vi "myRIO v1.0 DO Block Write.vi"(5 "Wait Until Done?":bool, 6 "DO FIFO Sample Rate (Hz)":dbl=1000.0 min=1000.0 max=8000000.0, 8 "error in (no error)":errorcluster, 9 "bool Value List":bool[][](array[boolean]), 10 "DO (N Samples) Channel List":T3, 11 "myRIO Ref In":T1) -> (0 "error out":errorcluster, 3 "myRIO Ref Out":T1)   [LabVIEW 2021]
uses:
  <vilib>/myRIO/Common/Instrument Driver Framework/myRIO v1.0/DO Block/typedefs/DO Block Channels List.ctl
  <vilib>/myRIO/Common/Instrument Driver Framework/myRIO v1.0/DO Block/typedefs/DO Block Channels Enum.ctl
  <vilib>/myRIO/Common/Instrument Driver Framework/Utilities/typedefs/myRIO v1.0 Reference.ctl
  <vilib>/myRIO/Common/Instrument Driver Framework/Utilities/typedefs/Generic FPGA Reference.ctl
  <vilib>/myRIO/Common/Instrument Driver Framework/myRIO v1.0/DO Block/typedefs/DO Block FPGA Reference.ctl
  <vilib>/myRIO/Common/Instrument Driver Framework/myRIO v1.0/DO Block/typedefs/DO Block Configuration.ctl
  <vilib>/myRIO/Common/Instrument Driver Framework/myRIO v1.0/Resource Manager/vis/myRIO v1.0 Block Write Configuration.vi
  <vilib>/rvi/errors/niLvFpgaAdjustHostInterfaceError.vi
  <vilib>/RVI Host/nirviSupport.llb/nirviErrorClusterFromErrorCode.vi
  <vilib>/rvi/interface/nirviReadWriteControl/nirviReadWriteControl.xnode
  <vilib>/rvi/interface/nirviMethod/nirviMethod.xnode
  <vilib>/rvi/interface/Simulation/niFpgaSimulationCallBeginRW.vi
  <vilib>/rvi/interface/nirviMethod/StockFPGA_InlinedMethodWaitForSingleIRQ.vi
  <vilib>/FPGAPlugInAG/Dynamic/niLvFpga_WaitOnIrq_Dynamic.vi
  <vilib>/FPGAPlugInAG/Dynamic/niLvFpga_AcknowledgeIrq_Dynamic.vi
  NiFpgaLv.dll
  <vilib>/FPGAPlugInAG/Dynamic/niLvFpga_WriteFifo_Dynamic.vi
  <vilib>/rvi/errors/niLvFpgaMergeErrorWithErrorCode.vi
panel:
  # "This VI writes boolean values to user specified a list of DIO channels on the myRIO v1.0 hardware. The values are input as boolean values. Please see Block Diagram for details."
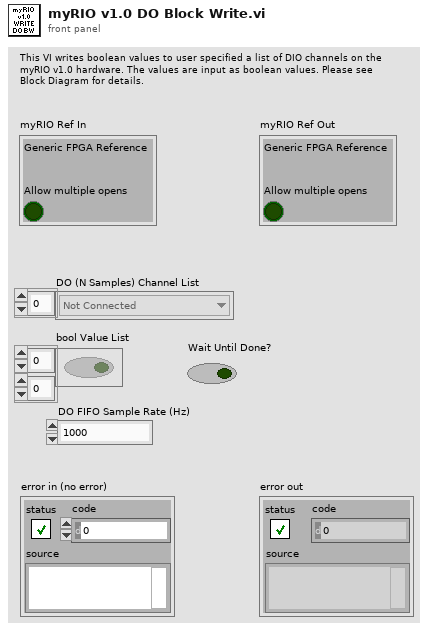
[diagram p1: front panel]
types:
  T1 = typedef "myRIO v1.0 Reference.ctl" = cluster{"Generic FPGA Reference":T2, "Allow multiple opens":bool}
  T2 = typedef "Generic FPGA Reference.ctl" = refnum<k20>
  T3 = typedef "DO Block Channels List.ctl" = T4[]
  T4 = typedef "DO Block Channels Enum.ctl" = enum16{"Not Connected", "A/DO0 (N Samples)", "A/DO1 (N Samples)", "A/DO2 (N Samples)", "A/DO3 (N Samples)", "A/DO4 (N Samples)", "A/DO5 (N Samples)", "A/DO6 (N Samples)", "A/DO7 (N Samples)", "A/DO8 (N Samples)", "A/DO9 (N Samples)", "A/DO10 (N Samples)", "A/DO11 (N Samples)", "A/DO12 (N Samples)", "A/DO13 (N Samples)", "A/DO14 (N Samples)", "A/DO15 (N Samples)", "A/DO16 (N Samples)", "A/DO17 (N Samples)", "A/DO18 (N Samples)", "A/DO19 (N Samples)", "B/DO0 (N Samples)", "B/DO1 (N Samples)", "B/DO2 (N Samples)", "B/DO3 (N Samples)", "B/DO4 (N Samples)", "B/DO5 (N Samples)", "B/DO6 (N Samples)", "B/DO7 (N Samples)", "B/DO8 (N Samples)", "B/DO9 (N Samples)", "B/DO10 (N Samples)", "B/DO11 (N Samples)", "B/DO12 (N Samples)", "B/DO13 (N Samples)", "B/DO14 (N Samples)", "B/DO15 (N Samples)", "B/DO16 (N Samples)", "B/DO17 (N Samples)", "B/DO18 (N Samples)", "B/DO19 (N Samples)"}
  T5 = typedef "DO Block FPGA Reference.ctl" = refnum<k20>
  T6 = typedef "DO Block Configuration.ctl" = cluster{"Wait Until Done?":bool, "DO FIFO Clock Divisor":u16, "Occurrence Handler":refnum<k4>, "Digital data reference":refnum<data-value>}
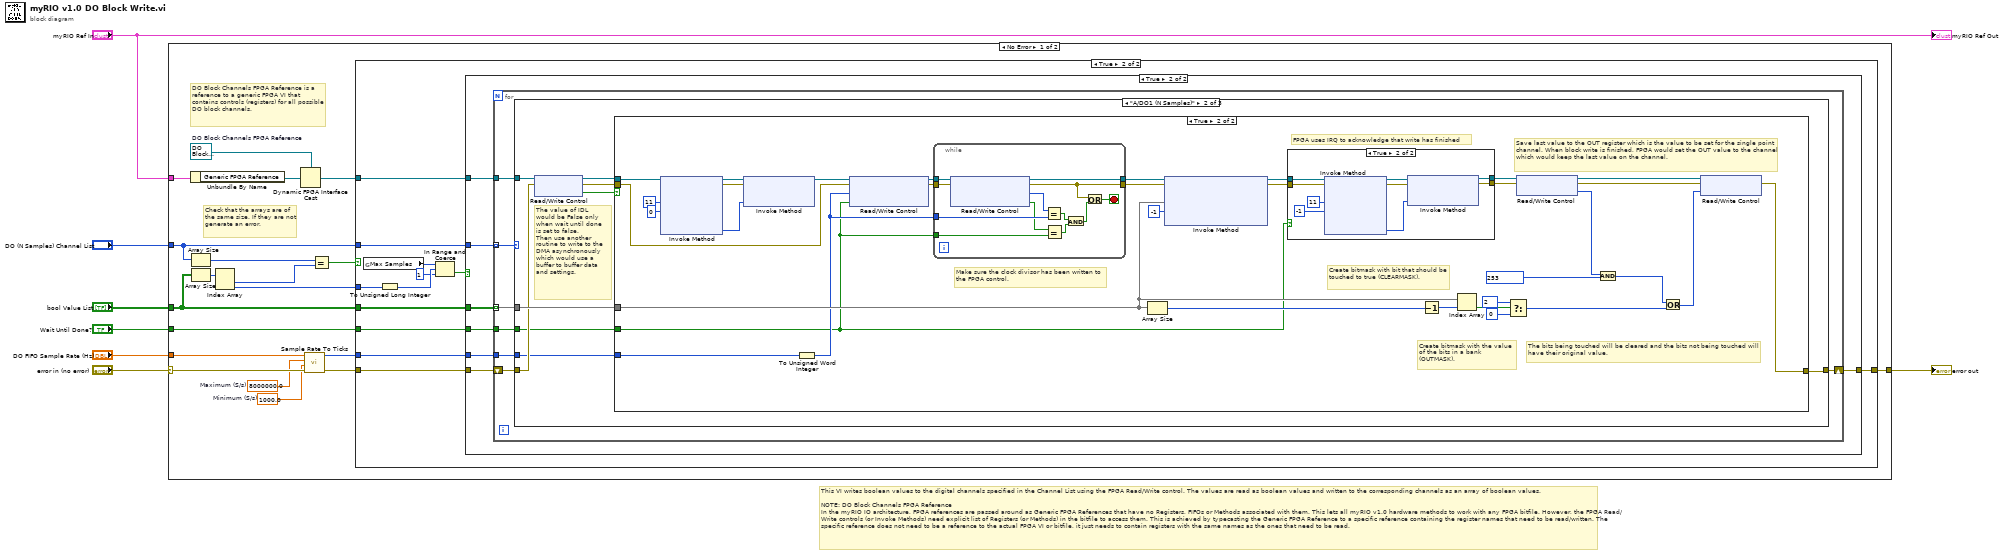
[diagram p0: block diagram]
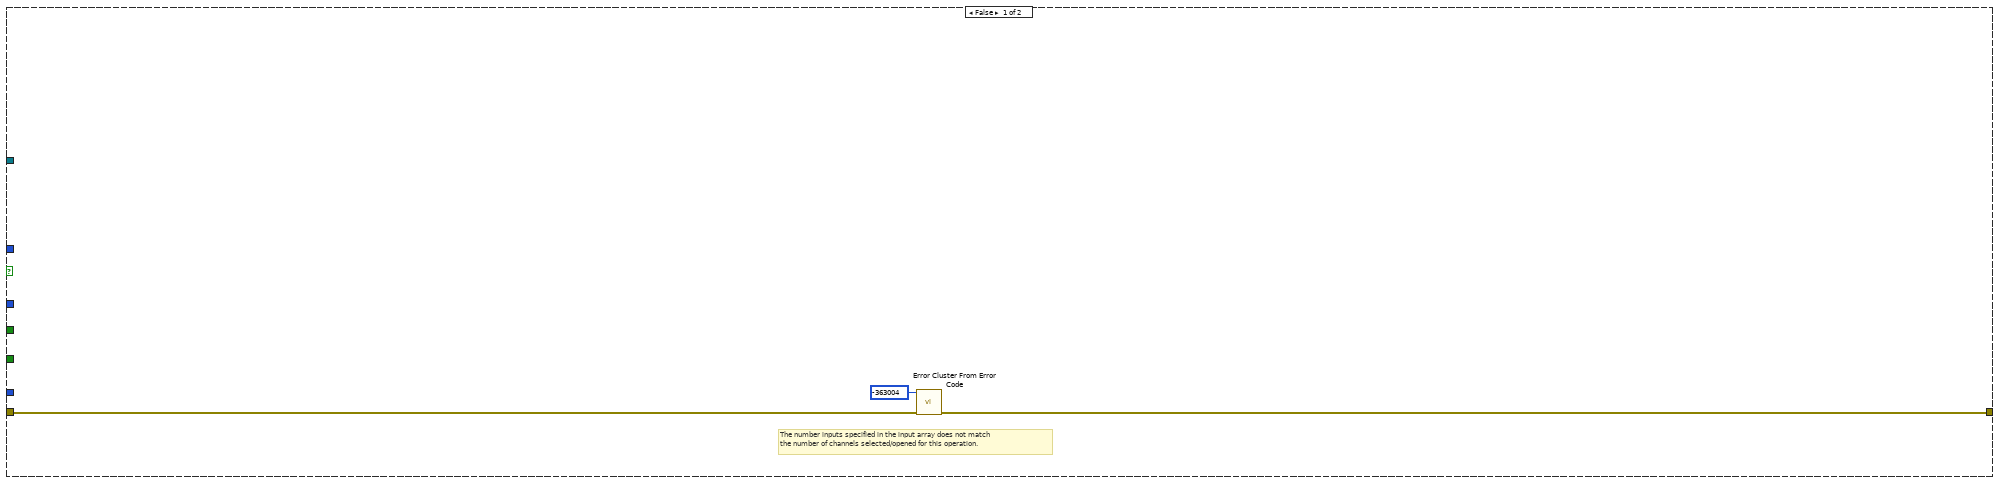
[diagram p2: hidden frame]
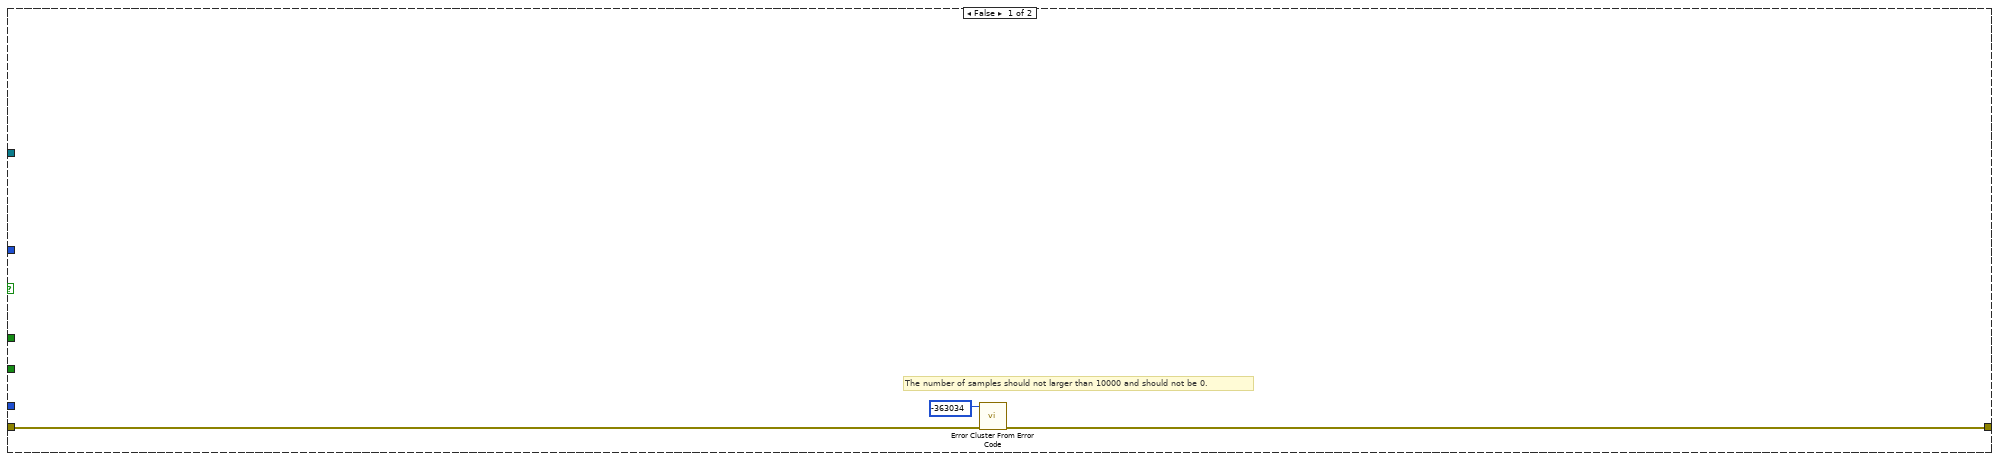
[diagram p3: hidden frame]
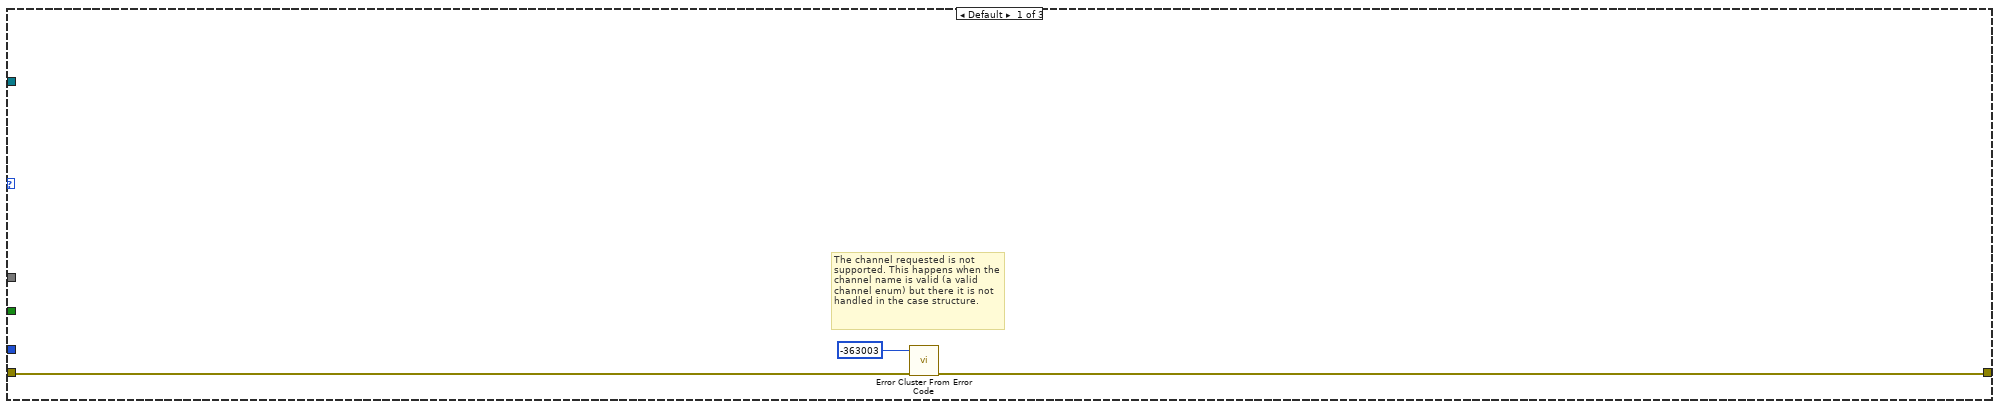
[diagram p4: hidden frame]
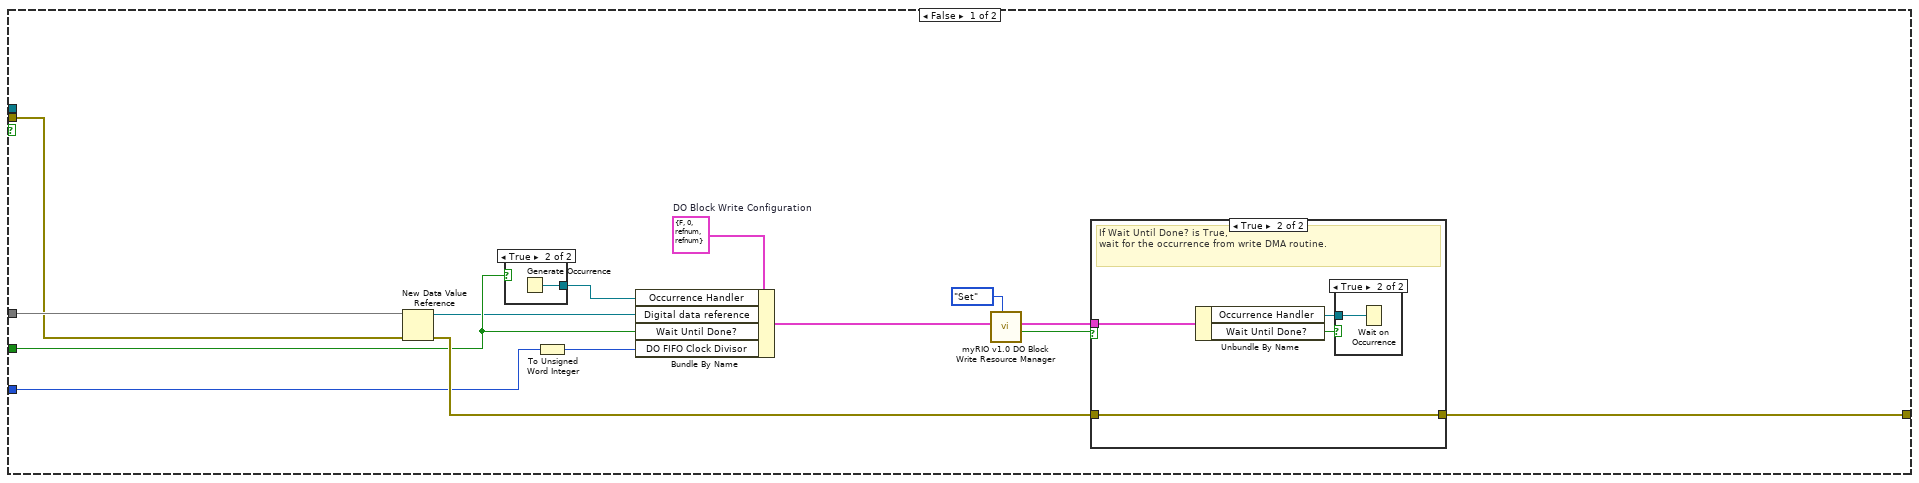
[diagram p5: hidden frame]
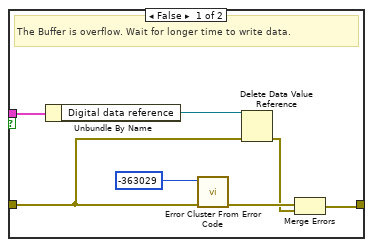
[diagram p6: hidden frame]
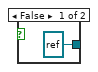
[diagram p8: hidden frame]
diagram:
  # "This VI writes boolean values to the digital channels specified in the Channel List using the FPGA Read/Write control. The values are read as boolean values and written to the corresponding channels as an array of boolean values. \n\nNOTE: DO Block Channels FPGA Reference\nIn the myRIO IO architecture, FPGA references are passed around as Generic FPGA References that have no Registers, FIFOs or Methods associated with them. This lets all myRIO v1.0 hardware methods to work with any FPGA bitfile. However, the FPGA Read/Write controls (or Invoke Methods) need explicit list of Registers (or Methods) in the bitfile to access them. This is achieved by typecasting the Generic FPGA Reference to a specific reference containing the register names that need to be read/written. The specific reference does not need to be a reference to the actual FPGA VI or bitfile, it just needs to contain registers with the same names as the ones that need to be read."
  n1 = case shown="No Error" "error in (no error)" {
    selector: "error in (no error)" -> [w10 w157]
    tunnel: "myRIO Ref In" -> [w26 _]
    tunnel: [w25 w157] -> w6
    tunnel: "DO (N Samples) Channel List" -> [w23 _]
    tunnel: "bool Value List" -> [w22 _]
    tunnel: "DO FIFO Sample Rate (Hz)" -> [w11 _]
    tunnel: "Wait Until Done?" -> [w18 _]
    frame No Error {
      w8 = 1000.0  # Minimum (S/s)
      w9 = 8000000.0  # Maximum (S/s)
      w17 = T5 refnum  # DO Block Channels FPGA Reference
      # "DO Block Channels FPGA Reference is a reference to a generic FPGA VI that contains controls (registers) for all possible DO block channels."
      # "Check that the arrays are of the same size. If they are not generate an error."
      n2 = Unbundle By Name(w26) -> ("Generic FPGA Reference"=w16:T2)
      n3 = Array Size(array=w23) -> (size(s)=w24:i32)
      n4 = Array Size(array=w22) -> (size(s)=w20:i32[])
      n5 = Index Array(array=w20) -> (element #1=w19:i32, element #2=w14:i32)  [unwired: 2 in]
      n6 = Dynamic FPGA Interface Cast(Session In=w17, Type=w16) -> (Session Out=w15:T5)
      n7 = call <vilib>:"Sample Rate To Ticks.vi"("error in (no error)"=w10, "Minimum (S/s)"=w8, "Maximum (S/s)"=w9, "Sample Rate (S/s)"=w11) -> ("error out"=w12:errorcluster, "Count (tick/s)"=w13:u32)  [unwired: 5 in, 1 out]
      n8 = Equal?(x=w24, y=w19) -> (x = y?=w21:bool)
      n9 = case shown="True" w21 {
        tunnel: w23 -> [_ w39]
        tunnel: w22 -> [_ w37]
        tunnel: w12 -> [w28 w41]
        tunnel: [w27 w40] -> w25
        tunnel: w13 -> [_ w38]
        tunnel: w18 -> [_ w34]
        tunnel: w15 -> [_ w36]
        tunnel: w14 -> [_ w35]
        frame False {
          # "The number inputs specified in the input array does not match\nthe number of channels selected/opened for this operation."
          n10 = call <vilib>:"Error Cluster From Error Code.vi"("error in (no error)"=w28, "error code (0)"=-363004) -> ("error out"=w27:errorcluster)  [unwired: 7 in]
        }
        frame True {
          n11 = global read "myRIO v1.0 Block Write Configuration.vi" "Max Samples"() -> (w32:u32)
          n12 = To Unsigned Long Integer(number=w35) -> (unsigned 32bit integer=w31:u32)
          n13 = In Range and Coerce(upper limit=w32, x=w31, lower limit=u32 1) -> (In Range?=w33:bool)  [unwired: 1 out]
          n14 = case shown="True" w33 {
            tunnel: w41 -> [w43 w51]
            tunnel: [w42 w50] -> w40
            tunnel: w39 -> [_ w49]
            tunnel: w38 -> [_ w48]
            tunnel: w37 -> [_ w47]
            tunnel: w36 -> [_ w46]
            tunnel: w34 -> [_ w45]
            frame False {
              # "The number of samples should not larger than 10000 and should not be 0."
              n15 = call <vilib>:"Error Cluster From Error Code.vi"("error in (no error)"=w43, "error code (0)"=-363034) -> ("error out"=w42:errorcluster)  [unwired: 7 in]
            }
            frame True {
              n16 = for {
                tunnel: w46 -> [w57]
                shift-right: [w53] -> w50
                shift-left: w51 -> [w56]
                tunnel: w49 -> [w58] mode=indexing
                tunnel: w48 -> [w55]
                tunnel: w47 -> [w54] mode=indexing
                tunnel: w45 -> [w52]
                n17 = case shown="\"A/DO1 (N Samples)\"" w58 {
                  tunnel: w57 -> [_ w66 _]
                  tunnel: w56 -> [w60 w65 w156]
                  tunnel: w55 -> [_ w62 _]
                  tunnel: w54 -> [_ w67 _]
                  tunnel: [w59 w64 w156] -> w53
                  tunnel: w52 -> [_ w63 _]
                  frame Default {
                    # "The channel requested is not supported. This happens when the channel name is valid (a valid channel enum) but there it is not handled in the case structure."
                    n18 = call <vilib>:"Error Cluster From Error Code.vi"("error in (no error)"=w60, "error code (0)"=-363003) -> ("error out"=w59:errorcluster)  [unwired: 7 in]
                  }
                  frame "A/DO1 (N Samples)" {
                    # "The value of IDL\nwould be False only \nwhen wait until done\nis set to false.\nThen use another \nroutine to write to the \nDMA asynchronously\nwhich would use a \nbuffer to buffer data \nand settings."
                    n19 = xnode "Read/Write Control"("FPGA VI Reference In"=w66, "error in"=w65) -> ("FPGA VI Reference Out"=w70:T5, "error out"=w69:errorcluster, "DO.A_1.IDL"=w68:bool)
                    n20 = case shown="True" w68 {
                      tunnel: w67 -> [w83 w111]
                      tunnel: [w79 w112] -> w64
                      tunnel: w70 -> [_ w103]
                      tunnel: w62 -> [w80 w110]
                      tunnel: w69 -> [w82 w101]
                      tunnel: w63 -> [w81 w99]
                      frame False {
                        w75 = T6 {"Wait Until Done?"=FALSE, "DO FIFO Clock Divisor"=0, "Occurrence Handler"=refnum, "Digital data reference"=refnum}  # DO Block Write Configuration
                        n21 = New Data Value Reference(data value=w83, error in=w82) -> (data value reference=w78:refnum<data-value>, error out=w84:errorcluster)
                        n22 = case shown="True" w81 {
                          tunnel: [refnum<k4> refnum ("occurrence") w98] -> w76
                          frame False {
                          }
                          frame True {
                            n23 = Generate Occurrence() -> (w98:refnum<k4>)
                          }
                        }
                        n24 = To Unsigned Word Integer(number=w80) -> (unsigned 16bit integer=w77:u16)
                        n25 = Bundle By Name(cluster=w75, "Occurrence Handler"=w76, "Digital data reference"=w78, "Wait Until Done?"=w81, "DO FIFO Clock Divisor"=w77) -> (w72:T6)
                        n26 = call <vilib>:"myRIO v1.0 DO Block Write Resource Manager.vi"("Action"=enum16{"Get", "Set"}."Set", "DO Resource In"=w72) -> ("Action Succeeds"=w73:bool, "DO Resource Out"=w71:T6)  [unwired: 8 in]
                        n27 = case shown="True" w73 {
                          tunnel: w84 -> [w88 w95]
                          tunnel: [w85 w95] -> w79
                          tunnel: w71 -> [w90 w92]
                          frame False {
                            # "The Buffer is overflow. Wait for longer time to write data."
                            n28 = Unbundle By Name(w90) -> ("Digital data reference"=w89:refnum<data-value>)
                            n29 = call <vilib>:"Error Cluster From Error Code.vi"("error in (no error)"=w88, "error code (0)"=-363029) -> ("error out"=w87:errorcluster)  [unwired: 7 in]
                            n30 = Delete Data Value Reference(data value reference=w89, error in=w88) -> (error out=w86:errorcluster)  [unwired: 1 out]
                            n31 = Merge Errors(w87, w86) -> (w85:errorcluster)
                          }
                          frame True {
                            # "If Wait Until Done? is True, \nwait for the occurrence from write DMA routine."
                            n32 = Unbundle By Name(w92) -> ("Occurrence Handler"=w93:refnum<k4>, "Wait Until Done?"=w94:bool)
                            n33 = case shown="True" w94 {
                              tunnel: w93 -> [_ w96]
                              frame False {
                              }
                              frame True {
                                n34 = Wait on Occurrence(2:w96) -> ()  [unwired: 2 in, 1 out]
                              }
                            }
                          }
                        }
                      }
                      frame True {
                        # "The bits being touched will be cleared and the bits not being touched will have their original value."
                        # "Make sure the clock divisor has been written to the FPGA control."
                        # "FPGA uses IRQ to acknowledge that write has finished"
                        # "Save last value to the OUT register which is the value to be set for the single point channel. When block write is finished, FPGA would set the OUT value to the channel which would keep the last value on the channel."
                        # "Create bitmask with the value of the bits in a bank (OUTMASK)."
                        # "Create bitmask with bit that should be touched to true (CLEARMASK)."
                        n35 = xnode "Invoke Method"("FPGA VI Reference In"=w103, "IRQ Number(s)"=11, "Timeout (ms)"=0) -> ("FPGA VI Reference Out"=w106:T5, "error out"=w105:errorcluster, "IRQ(s) Asserted"=w104:i32)  [unwired: 1 in, 1 out]
                        n36 = xnode "Invoke Method"("FPGA VI Reference In"=w106, "error in"=w105, "IRQ Number(s)"=w104) -> ("FPGA VI Reference Out"=w102:T5)  [unwired: 1 out]
                        n37 = To Unsigned Word Integer(number=w110) -> (unsigned 16bit integer=w109:u16)
                        n38 = xnode "Read/Write Control"("FPGA VI Reference In"=w102, "error in"=w101, "DO.A_1.ClockDivisor"=w109, "DO.A_1.IRQ.SELECT"=w99) -> ("FPGA VI Reference Out"=w132:T5, "error out"=w131:errorcluster)
                        n39 = while {
                          tunnel: w132 -> [w155]
                          tunnel: [w154] -> w117
                          tunnel: [w149] -> w116
                          tunnel: w131 -> [w153]
                          tunnel: w109 -> [w152]
                          tunnel: w99 -> [w147]
                          stop <- w150 stop-if-true
                          n40 = xnode "Read/Write Control"("FPGA VI Reference In"=w155, "error in"=w153) -> ("FPGA VI Reference Out"=w154:T5, "error out"=w149:errorcluster, "DO.A_1.ClockDivisor"=w151:u16, "DO.A_1.IRQ.SELECT"=w148:bool)
                          n41 = Equal?(x=w151, y=w152) -> (x = y?=w146:bool)
                          n42 = Equal?(x=w148, y=w147) -> (x = y?=w145:bool)
                          n43 = And(x=w146, y=w145) -> (x .and. y?=w144:bool)
                          n44 = Or(x=w149, y=w144) -> (x .or. y?=w150:bool)
                        }
                        n45 = Array Size(array=w111) -> (size(s)=w100:i32)
                        n46 = xnode "Invoke Method"("FPGA VI Reference In"=w117, "error in"=w116, "Data"=w111, "Timeout (ms)"=-1) -> ("FPGA VI Reference Out"=w119:T5, "error out"=w118:errorcluster)  [unwired: 1 out]
                        n47 = case shown="True" w99 {
                          tunnel: w119 -> [w133 w142]
                          tunnel: w118 -> [w134 w141]
                          tunnel: [w134 w137] -> w113
                          tunnel: [w133 w136] -> w114
                          frame False {
                          }
                          frame True {
                            n48 = xnode "Invoke Method"("FPGA VI Reference In"=w142, "error in"=w141, "IRQ Number(s)"=11, "Timeout (ms)"=-1) -> ("FPGA VI Reference Out"=w140:T5, "error out"=w139:errorcluster, "IRQ(s) Asserted"=w138:i32)  [unwired: 1 out]
                            n49 = xnode "Invoke Method"("FPGA VI Reference In"=w140, "error in"=w139, "IRQ Number(s)"=w138) -> ("FPGA VI Reference Out"=w136:T5, "error out"=w137:errorcluster)
                          }
                        }
                        n50 = Decrement(x=w100) -> (x-1=w115:i32)
                        n51 = Index Array(array=w111, index=w115) -> (element=w129:bool)
                        n52 = Select(t=u8 2 ("y"), s=w129, f=u8 0 ("y")) -> (s? t:f=w120:u8)
                        n53 = xnode "Read/Write Control"("FPGA VI Reference In"=w114, "error in"=w113) -> ("FPGA VI Reference Out"=w126:T5, "error out"=w125:errorcluster, "DIO.A_7:0.OUT"=w124:u8)
                        n54 = And(x=w124, y=u8 253) -> (x .and. y?=w123:u8)
                        n55 = Or(x=w123, y=w120) -> (x .or. y?=w122:u8)
                        n56 = xnode "Read/Write Control"("FPGA VI Reference In"=w126, "error in"=w125, "DIO.A_7:0.OUT"=w122) -> ("error out"=w112:errorcluster)  [unwired: 1 out]
                      }
                    }
                  }
                  frame "Not Connected" {
                  }
                }
              }
            }
          }
        }
      }
    }
    frame Error {
    }
  }
  "error out" <- w6
  "myRIO Ref Out" <- "myRIO Ref In"
